vi "vision v4.vi"(0 "Image In":T1, 7 "error in":errorcluster) -> (20 "Image Out":T1, 27 "error out":errorcluster)   [LabVIEW 2016]
uses:
  <vilib>/vision/Image Controls.llb/IMAQ Image.ctl
  <vilib>/vision/NI_Vision_Development_Module.lvlib
panel:
  in  "Blue or Luma or Val or Inten Range":cluster{"Lower value":i32, "Upper value":i32}={"Lower value"=50, "Upper value"=255}
  in  "Green or Sat Range":cluster{"Lower value":i32, "Upper value":i32}={"Lower value"=30, "Upper value"=255}
  in  "Red or Hue Range":cluster{"Lower value":i32, "Upper value":i32}={"Lower value"=80, "Upper value"=170}
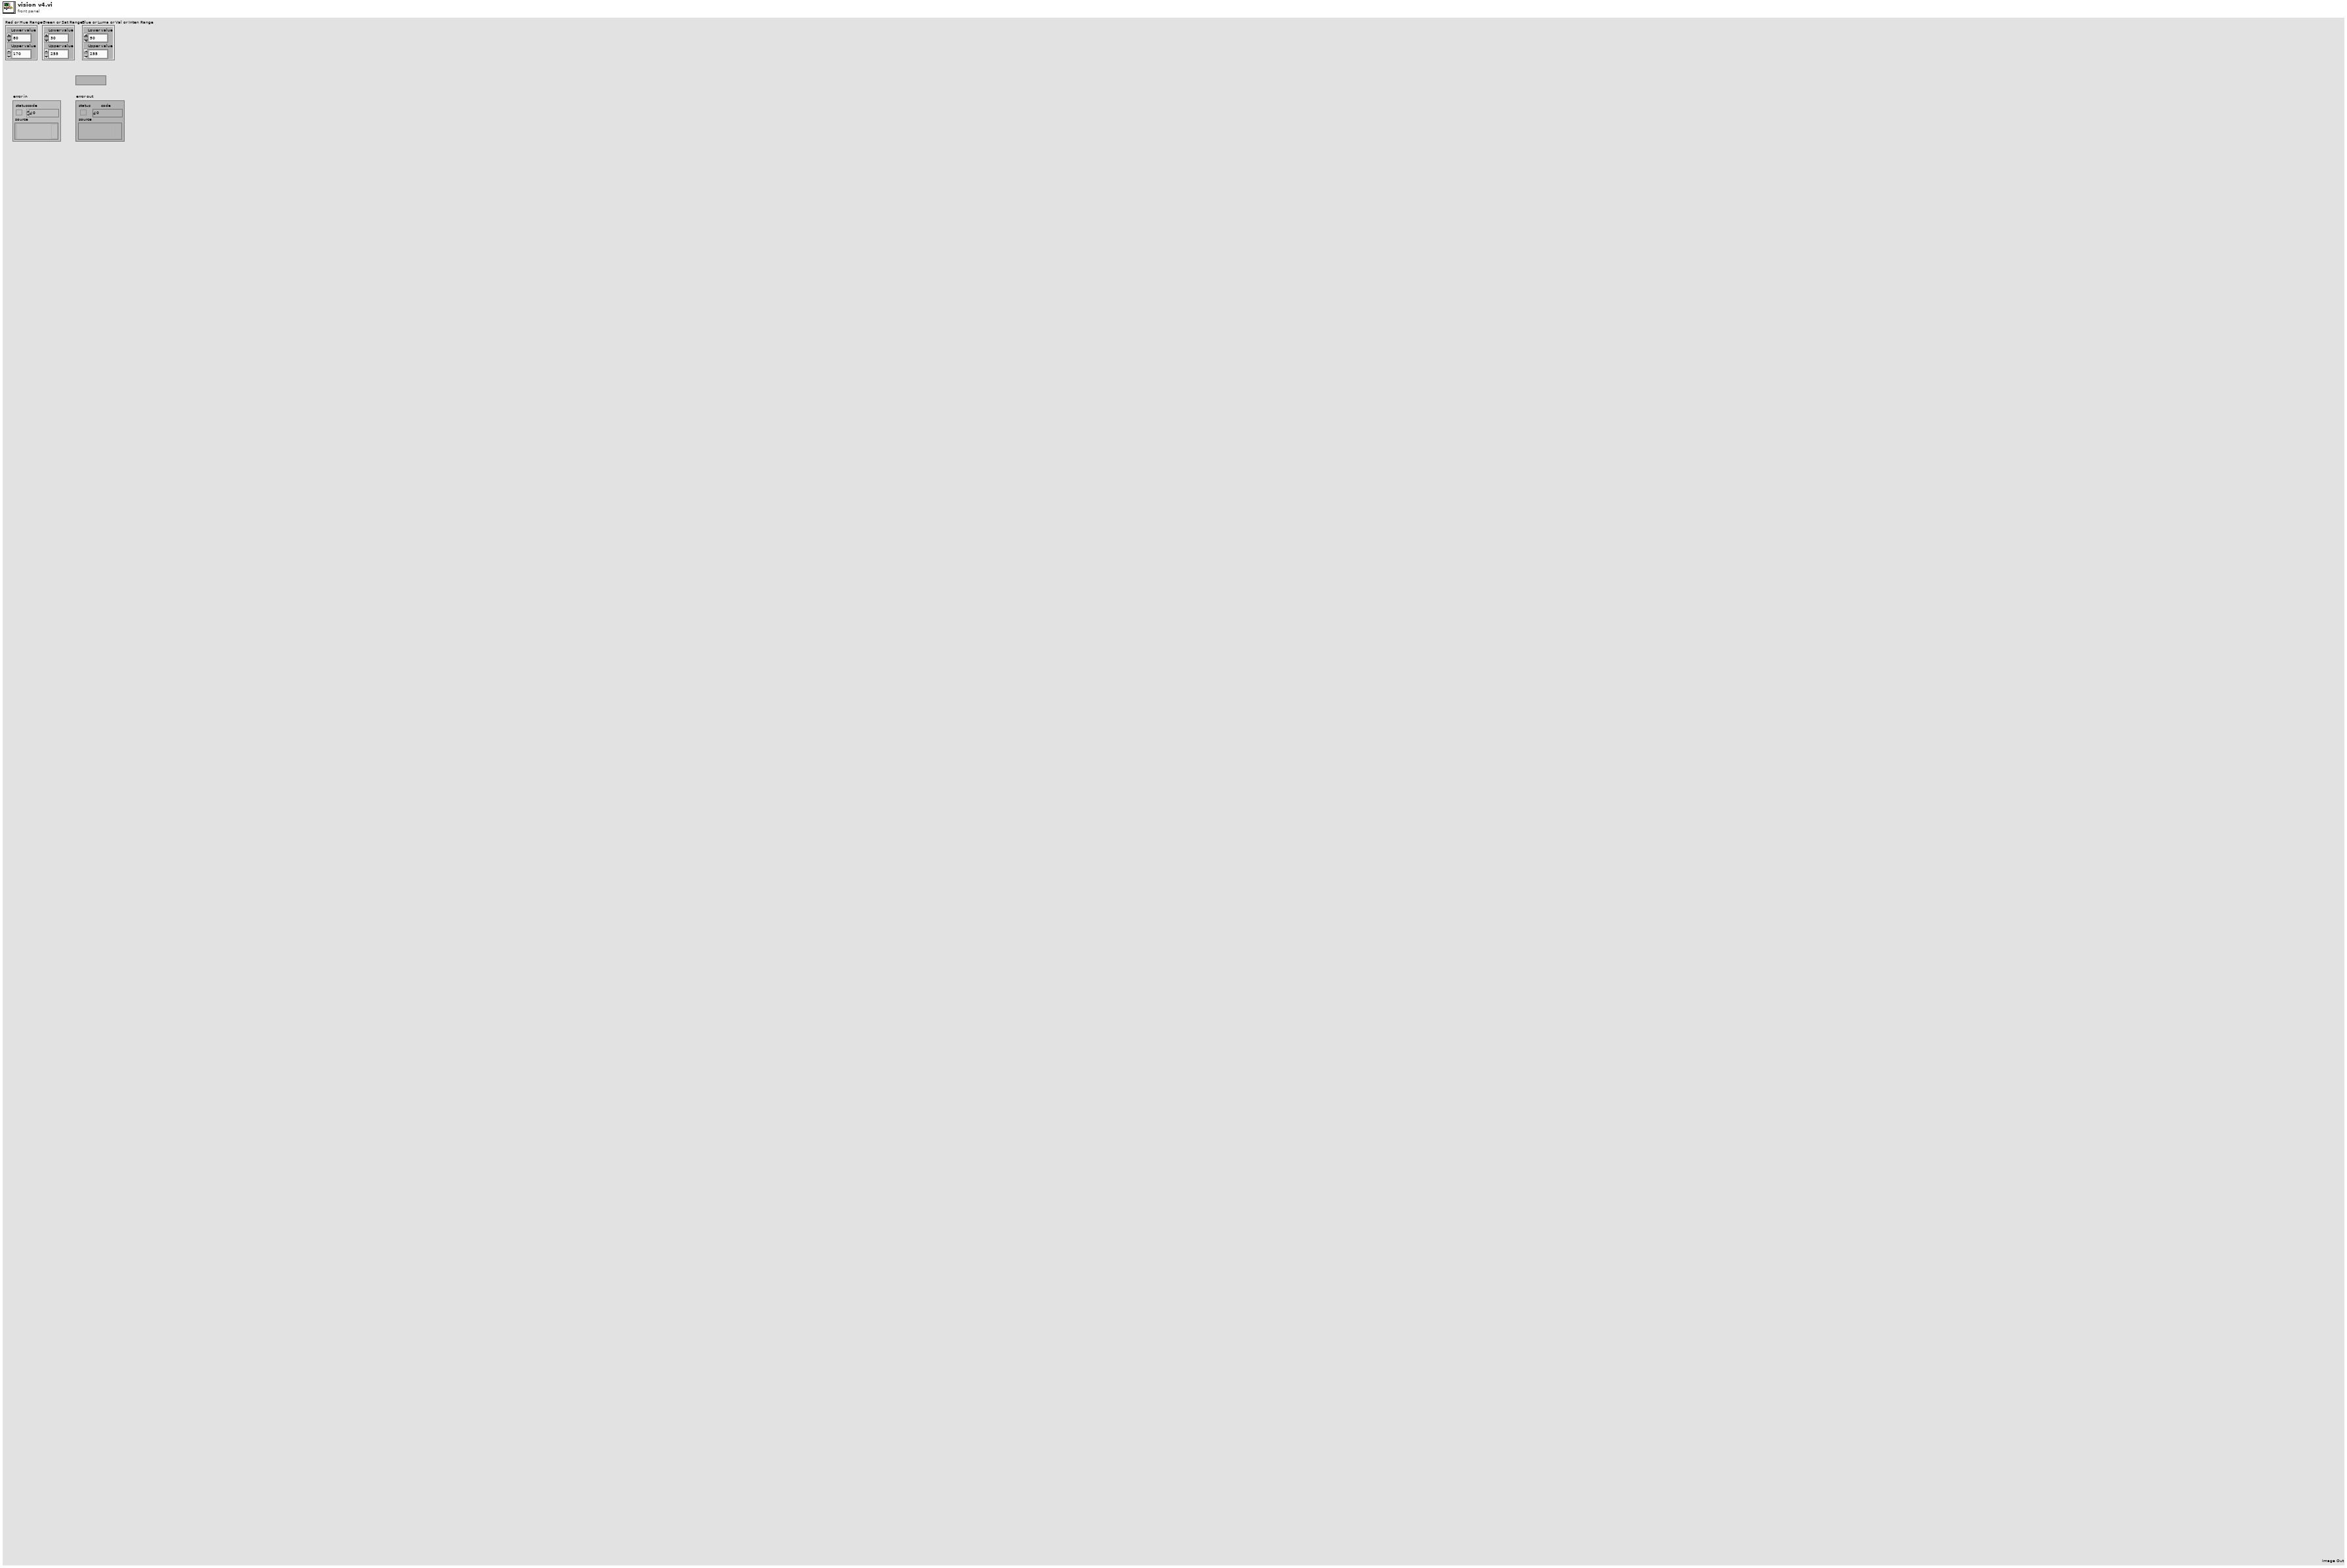
[diagram p1: front panel]
types:
  T1 = typedef "IMAQ Image.ctl" = refnum<image>
  T2 = cluster{"Measurement Parameter":i32, "Range Lower Value":dbl, "Range Upper Value":dbl, "Range":bool, "Measurement Type":bool}[]
  T3 = enum32{"AutoM", "Close", "Dilate", "Erode", "Gradient", "Gradient out", "Gradient in", "Hit miss", "Open", "PClose", "POpen", "Thick", "Thin"}
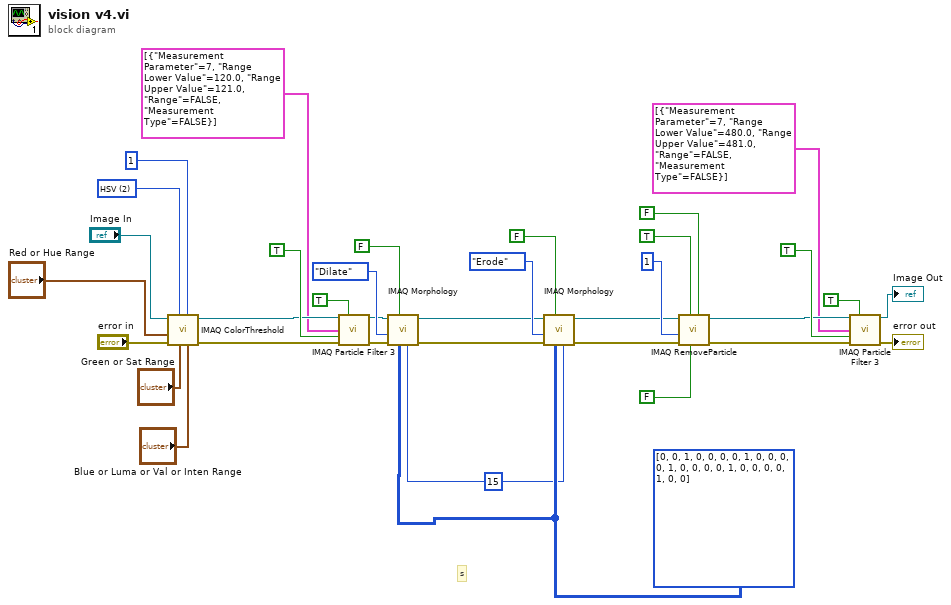
[diagram p0: block diagram]
diagram:
  w1 = 15 ("Number of iterations (1)")
  w2 = i32[][] [[0, 0, 1, 0, 0], [0, 0, 1, 0, 0], [0, 0, 1, 0, 0], [0, 0, 1, 0, 0], [0, 0, 1, 0, 0]] ("Structuring Element")
  w34 = u16 2 items=["RGB", "HSL", "HSV", "HSI"] ("Color Mode")
  # "s"
  n1 = call "IMAQ ColorThreshold"("Blue or Luma or Val or Inten Range"="Blue or Luma or Val or Inten Range", "Replace Value"=1, "Green or Sat Range"="Green or Sat Range", "Color Mode"=w34, "error in (no error)"="error in", "Red or Hue Range"="Red or Hue Range", "Image Src"="Image In") -> ("error out"=w25:errorcluster, "Image Dst Out"=w26:T1)  [unwired: 1 in, 2 out]
  n2 = call "IMAQ Particle Filter 3"("Image Src"=w26, "Connectivity 4/8 (8)"=TRUE, "Selection Values"=T2 [{"Measurement Parameter"=7, "Range Lower Value"=120.0, "Range Upper Value"=121.0, "Range"=FALSE, "Measurement Type"=FALSE}], "Keep/Remove Particles (F)"=TRUE ("Keep/Remove Particles"), "error in (no error)"=w25) -> ("Image Dst Out"=w21:T1, "error out"=w20:errorcluster)  [unwired: 4 in, 5 out]
  n3 = call "IMAQ Morphology"("Number of iterations (1)"=w1, "Structuring Element"=w2, "Square/Hexa (Square)"=FALSE, "error in (no error)"=w20, "Operation"=T3."Dilate", "Image Src"=w21) -> ("error out"=w16:errorcluster, "Image Dst Out"=w17:T1)  [unwired: 1 in, 3 out]
  n4 = call "IMAQ Morphology"("Number of iterations (1)"=w1, "Structuring Element"=w2, "Square/Hexa (Square)"=FALSE, "error in (no error)"=w16, "Operation"=T3."Erode", "Image Src"=w17) -> ("error out"=w10:errorcluster, "Image Dst Out"=w11:T1)  [unwired: 1 in, 3 out]
  n5 = call "IMAQ RemoveParticle"("Connectivity 4/8 (8)"=FALSE, "Low Pass/High Pass (Low)"=FALSE, "Square/Hexa (Square)"=TRUE, "error in (no error)"=w10, "Number of Erosion"=1, "Image Src"=w11) -> ("error out"=w4:errorcluster, "Image Dst Out"=w5:T1)  [unwired: 1 in, 3 out]
  n6 = call "IMAQ Particle Filter 3"("Image Src"=w5, "Connectivity 4/8 (8)"=TRUE, "Selection Values"=T2 [{"Measurement Parameter"=7, "Range Lower Value"=480.0, "Range Upper Value"=481.0, "Range"=FALSE, "Measurement Type"=FALSE}], "Keep/Remove Particles (F)"=TRUE ("Keep/Remove Particles"), "error in (no error)"=w4) -> ("Image Dst Out"=→"Image Out":T1, "error out"=→"error out":errorcluster)  [unwired: 4 in, 5 out]
